vi "Add Font to Stylesheet.vi"(8 "error in":errorcluster, 10 "Font in":refnum<k24>, 11 "SpreadsheetDoc in":refnum<k24>) -> (0 "error out":errorcluster, 1 "Index":i32, 2 "Font out":refnum<k24>, 3 "SpreadsheetDoc out":refnum<k24>)   [LabVIEW 2021, in "Open Xml.lvlib"]
uses:
  Open Xml.lvlib
  D:/git/Open-Xml-LabVIEW/dll/DocumentFormat.OpenXml.dll
  dll/DocumentFormat.OpenXml.dll
  D:/git/Open-Xml-LabVIEW/dll/DocumentFormat.OpenXml.Framework.dll
  dll/DocumentFormat.OpenXml.Framework.dll
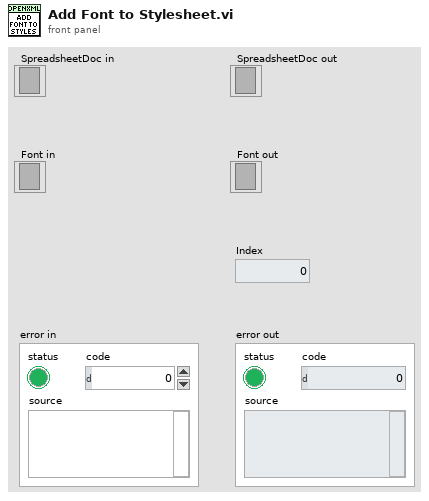
[diagram p1: front panel]
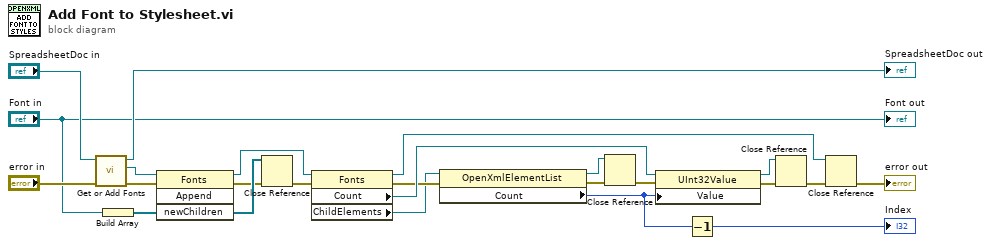
[diagram p0: block diagram]
diagram:
  n1 = call "Get or Add Fonts.vi"("error in"="error in", "SpreadsheetDoc in"="SpreadsheetDoc in") -> ("error out"=w22:errorcluster, "Fonts"=w20:refnum<k24>, "SpreadsheetDoc out"=→"SpreadsheetDoc out":refnum<k24>)  [unwired: 7 in]
  n2 = Build Array("Font in") -> (w7:refnum<k24>[])
  n3 = invoke class="Fonts" method="Append"(reference=w20, error in=w22, "newChildren"=w7) -> (reference out=w18:refnum<k24>, error out=w5:errorcluster, "newChildren"=w6:refnum<k24>[])  [unwired: 1 in, 1 out]
  n4 = Close Reference(reference=w6, error in (no error)=w5) -> (error out=w1:errorcluster)
  n5 = property class="Fonts"(reference=w18, error in=w1) -> (reference out=w17:refnum<k24>, error out=w12:errorcluster, "Count"=w16:refnum<k24>, "ChildElements"=w11:refnum<k24>)
  n6 = property class="OpenXmlElementList"(reference=w11, error in=w12) -> (reference out=w3:refnum<k24>, error out=w10:errorcluster, "Count"=w9:i32)
  n7 = Close Reference(reference=w3, error in (no error)=w10) -> (error out=w4:errorcluster)
  n8 = property class="UInt32Value"(reference=w16, error in=w4, "Value"=w9) -> (reference out=w13:refnum<k24>, error out=w15:errorcluster)
  n9 = Decrement(x=w9) -> (x-1=→"Index":i32)
  n10 = Close Reference(reference=w13, error in (no error)=w15) -> (error out=w14:errorcluster)
  n11 = Close Reference(reference=w17, error in (no error)=w14) -> (error out=→"error out":errorcluster)
  "Font out" <- "Font in"
